vi "HTTP下载文件.vi"   [LabVIEW 2016]
types:
  T1 = enum16{"open", "replace", "create", "open or create", "replace or create", "replace or create with confirmation"}
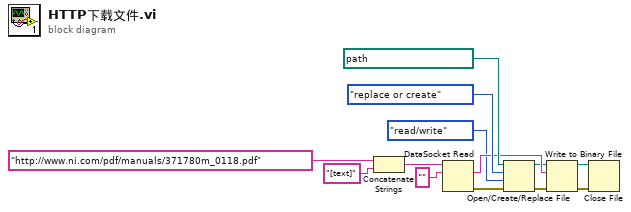
[diagram p0: block diagram]
diagram:
  n1 = Concatenate Strings("http://www.ni.com/pdf/manuals/371780m_0118.pdf", "[text]" ("字符串")) -> (w11:string)
  n2 = DataSocket Read(10:"", 11:w11) -> (0:w6:errorcluster, 2:w7:string)  [unwired: 3 in, 5 out]
  n3 = Open/Create/Replace File(file path (use dialog)=path "D:/2106升级说明.pdf" ("文件（使用对话框）"), error in=w6, operation (0:open)=T1."replace or create" ("操作(0:open)"), access (0:read/write)=enum16{"read/write", "read-only", "write-only"}."read/write" ("权限(0:read/write)")) -> (refnum out=w4:refnum<file>, error out=w5:errorcluster)  [unwired: 2 in, 1 out]
  n4 = Write to Binary File(file (use dialog)=w4, data=w7, error in=w5) -> (refnum out=w1:refnum<file>, error out=w2:errorcluster)  [unwired: 3 in, 1 out]
  n5 = Close File(refnum=w1, error in=w2) -> ()  [unwired: 2 out]
